vi "extract FFT matrix fix B.vi"(5 "B index":i32, 7 "all field rows":dbl[][](array[numeric]), 10 "parameter":dbl[][](array[numeric]), 11 "all data rows":dbl[][](array[numeric])) -> (2 "plot parameter":T1, 3 "FFT matrix":dbl[][](array[numeric]))   [LabVIEW 2021]
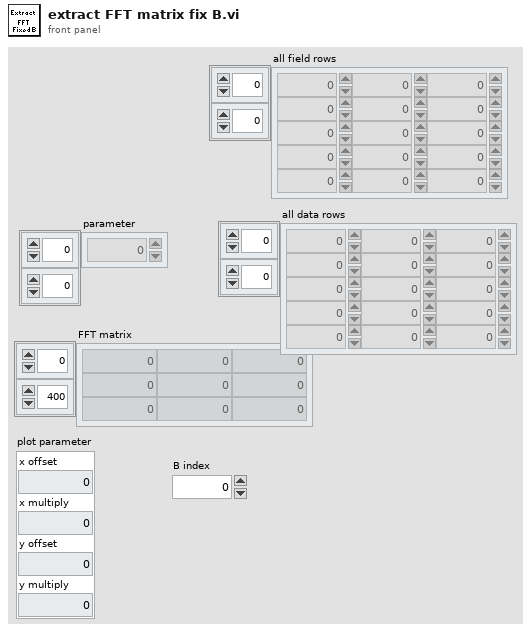
[diagram p1: front panel]
types:
  T1 = cluster{"x offset":dbl, "x multiply":dbl, "y offset":dbl, "y multiply":dbl}
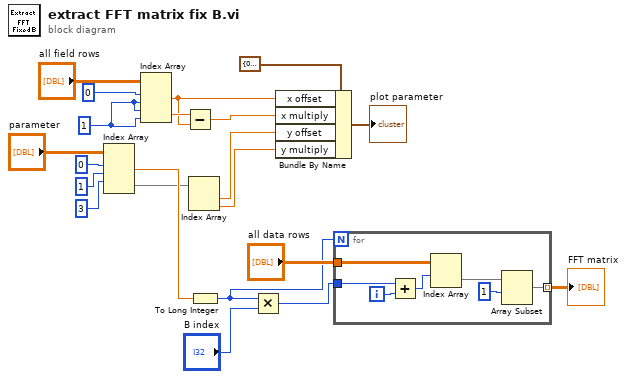
[diagram p0: block diagram]
diagram:
  w1 = 1 ("disabled index (col)")
  n1 = Index Array(array="parameter", index (row) #1=0 ("index (row)"), index (col) #1=1 ("disabled index (col)"), index (row) #2=3 ("index (row)")) -> (element #1=w8:dbl, element #2=w2:dbl[])  [unwired: 1 in]
  n2 = Index Array(array="all field rows", index (row) #1=0 ("index (row)"), index (col) #1=w1, index (row) #2=w1, index (col) #2=w1) -> (element #1=w14:dbl, element #2=w15:dbl)
  n3 = Subtract(x=w15, y=w14) -> (x-y=w13:dbl)
  n4 = Index Array(array=w2) -> (element #1=w12:dbl, element #2=w11:dbl)  [unwired: 2 in]
  n5 = To Long Integer(number=w8) -> (32bit integer=w7:i32)
  n6 = Multiply(x=w7, y="B index") -> (x*y=w5:i32)
  n7 = Bundle By Name(cluster=T1 {"x offset"=0.0, "x multiply"=0.0, "y offset"=0.0, "y multiply"=0.0} ("plot parameter"), "x offset"=w14, "x multiply"=w13, "y offset"=w12, "y multiply"=w11) -> (→"plot parameter":T1)
  n8 = for {
    N: w7 -> [_]
    tunnel: "all data rows" -> [w28]
    tunnel: [w25] -> w18 mode=indexing
    tunnel: w5 -> [w24]
    i -> [w23]
    n9 = Add(x=w24, y=w23) -> (x+y=w22:i32)
    n10 = Index Array(array=w28, index (row)=w22) -> (element=w27:dbl[])  [unwired: 1 in]
    n11 = Array Subset(array=w27, index=1) -> (w25:dbl[])  [unwired: 1 in]
  }
  "FFT matrix" <- w18
